vi "ReadDefaultConfigFile.vi"(8 "error in (no error)":errorcluster, 11 "SMO.UI.MAUI in":refnum<class "SMO.UI.MAUI.lvclass">) -> (0 "error out":errorcluster, 2 "Default Data":T1={"Default Subpanel Path"="\\templates\\JKI\\JKI SMO\\LevyLab\\SMO.UI.Embedded.Basic.lvclass"}, 3 "SMO.UI.MAUI out":refnum<class "SMO.UI.MAUI.lvclass">)   [LabVIEW 2020, in "SMO.UI.MAUI.lvclass"]
uses:
  SMO.UI.MAUI.lvclass
  Typedefs/DefaultConfiguration.ctl
  <vilib>/addons/_JKI.lib/Serialization/JSON/JKI JSON Serialization.lvlib
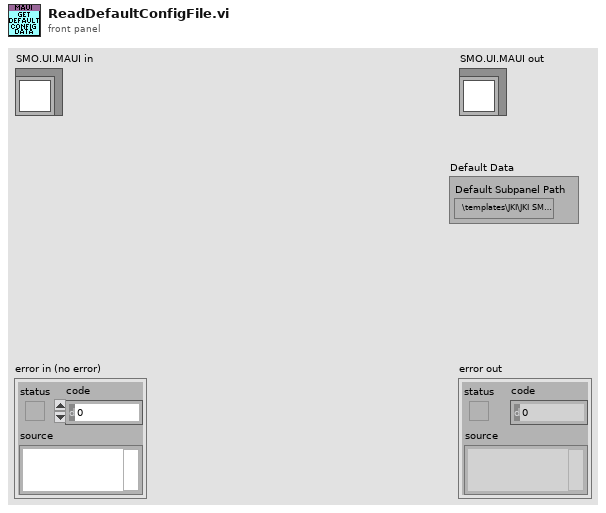
[diagram p1: front panel]
types:
  T1 = typedef "SMO.UI.MAUI.lvclass/DefaultConfiguration.ctl" = cluster{"Default Subpanel Path":string}
  T2 = enum16{"open", "replace", "create", "open or create", "replace or create", "replace or create with confirmation"}
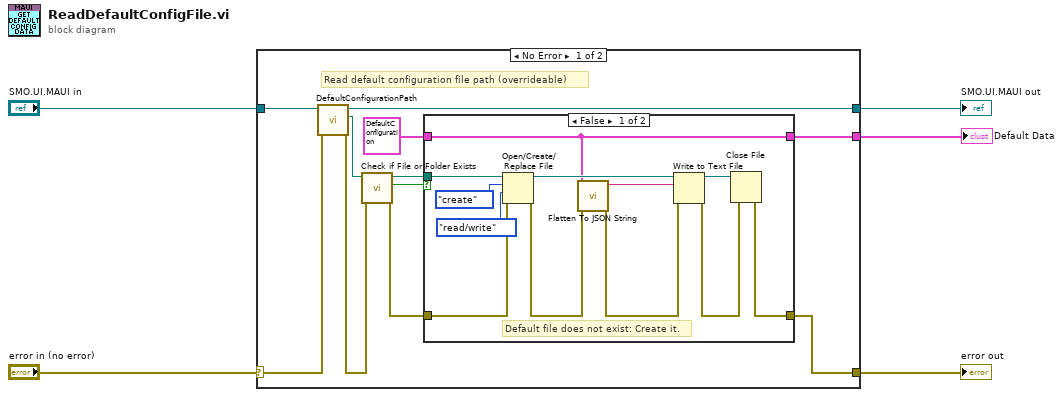
[diagram p0: block diagram]
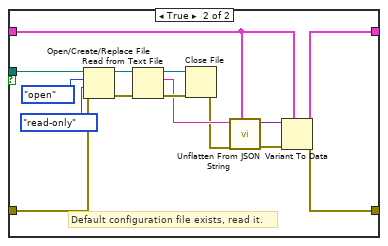
[diagram p2: hidden frame]
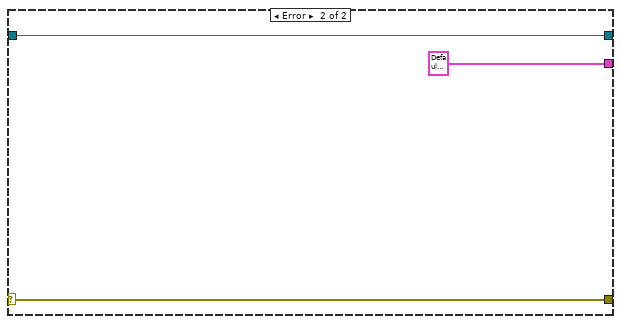
[diagram p3: hidden frame]
diagram:
  n1 = case shown="No Error" "error in (no error)" {
    selector: "error in (no error)" -> [w11 w46]
    tunnel: [w6 w46] -> w4
    tunnel: [w8 w45] -> w2
    tunnel: "SMO.UI.MAUI in" -> [w9 w45]
    tunnel: [w7 T1 {"Default Subpanel Path"="\\templates\\JKI\\JKI SMO\\LevyLab\\SMO.UI.Embedded.Basic.lvclass"} ("Default Data")] -> w1
    frame No Error {
      # "Read default configuration file path (overrideable)"
      n2 = call-dynamic "DefaultConfigurationPath.vi"("error in (no error)"=w11, "SMO.UI.MAUI in"=w9) -> ("error out"=w15:errorcluster, "Path"=w16:path, "SMO.UI.MAUI out"=w8:refnum<class "SMO.UI.MAUI.lvclass">)  [unwired: 7 in]
      n3 = call <vilib>:"Check if File or Folder Exists.vi"("error in (no error)"=w15, "path"=w16) -> ("error out"=w10:errorcluster, "file or folder exists?"=w14:bool, "dup path"=w13:path)  [unwired: 7 in]
      n4 = case shown="False" w14 {
        tunnel: w13 -> [w26 w43]
        tunnel: w10 -> [w23 w42]
        tunnel: T1 {"Default Subpanel Path"="templates\\JKI\\JKI SMO\\LevyLab\\SMO.UI.Embedded.Basic.lvclass"} ("Default Data") -> [w17 w31]
        tunnel: [w18 w30] -> w6
        tunnel: [w17 w29] -> w7
        frame False {
          # "Default file does not exist: Create it."
          n5 = Open/Create/Replace File(file path (use dialog)=w26, error in=w23, operation (0:open)=T2."create", access (0:read/write)=enum16{"read/write", "read-only", "write-only"}."read/write") -> (refnum out=w25:refnum<file>, error out=w22:errorcluster)  [unwired: 2 in, 1 out]
          n6 = call <vilib>:"Flatten To JSON String.vi"("error in (no error)"=w22, "Variant"=w17) -> ("error out"=w19:errorcluster, "JSON String"=w24:string)  [unwired: 8 in]
          n7 = Write to Text File(file (use dialog)=w25, text=w24, error in=w19) -> (refnum out=w20:refnum<file>, error out=w21:errorcluster)  [unwired: 1 in, 1 out]
          n8 = Close File(refnum=w20, error in=w21) -> (error out=w18:errorcluster)  [unwired: 1 out]
        }
        frame True {
          # "Default configuration file exists, read it."
          n9 = Open/Create/Replace File(file path (use dialog)=w43, error in=w42, operation (0:open)=T2."open", access (0:read/write)=enum16{"read/write", "read-only", "write-only"}."read-only") -> (refnum out=w39:refnum<file>, error out=w38:errorcluster)  [unwired: 2 in, 1 out]
          n10 = Read from Text File(file (use dialog)=w39, error in=w38) -> (refnum out=w37:refnum<file>, text=w35:string, error out=w36:errorcluster)  [unwired: 2 in, 1 out]
          n11 = Close File(refnum=w37, error in=w36) -> (error out=w32:errorcluster)  [unwired: 1 out]
          n12 = call <vilib>:"Unflatten From JSON String.vi"("Type and Defaults"=w31, "error in (no error)"=w32, "JSON String"=w35) -> ("error out"=w33:errorcluster, "Variant"=w34:variant)  [unwired: 7 in]
          n13 = Variant To Data(error in=w33, type=w31, Variant=w34) -> (data=w29:T1, error out=w30:errorcluster)
        }
      }
    }
    frame Error {
    }
  }
  "error out" <- w4
  "SMO.UI.MAUI out" <- w2
  "Default Data" <- w1
